vi "AdditionalInfoManupulation.vi"(8 "error in":errorcluster, 10 "Remarks":string, 11 "Temperature":dbl) -> (0 "error out":errorcluster, 3 "Additional Info":T1)   [LabVIEW 2018]
uses:
  Controls/AdditionalData.ctl
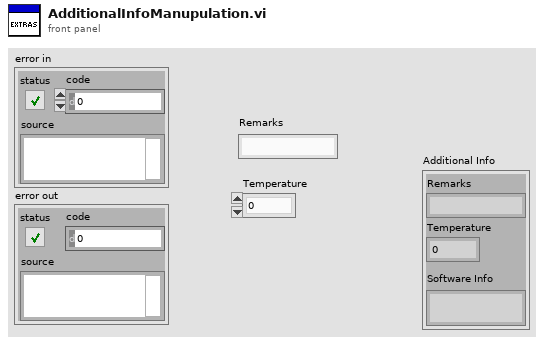
[diagram p1: front panel]
types:
  T1 = typedef "AdditionalData.ctl" = cluster{"Remarks":string, "Temperature":dbl, "Software Info":string}
  T2 = cluster{"Remarks":string, "Temperature":dbl, string}
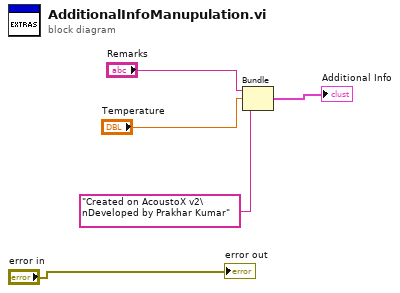
[diagram p0: block diagram]
diagram:
  n1 = Bundle("Remarks"="Remarks", "Temperature"="Temperature", "Created on AcoustoX v2\nDeveloped by Prakhar Kumar") -> (→"Additional Info":T2)  [unwired: 1 in]
  "error out" <- "error in"
